vi "masternslave.vi"() -> ()   [LabVIEW 2020]
panel:
  in  "Requested Configuration (2: Query)":u32(ring)=2 items=["Off", "On", "Query"]
  out "Target Power Enabled?":bool
  in  "stop":bool
  out "Actual Bitrate kHz":i32=1000
  in  "Requested Bitrate kHz (1000)":i32=1000 min=0 max=50000
  out "Unique Ids":u32[](array[numeric])
  out "Data In":u8[](array[numeric]) format="%.0x"
  out "Total Shifted Out":i32
  in  "Max Bytes to Retrieve (256)":u32=256 min=1
  out "Batch Length":i32
  in  "Data Out (none)":u32[](array[numeric]) format="%.0x"
  in  "Output Enable (on)":bool=TRUE
  out "Ports":u16[](array[numeric])
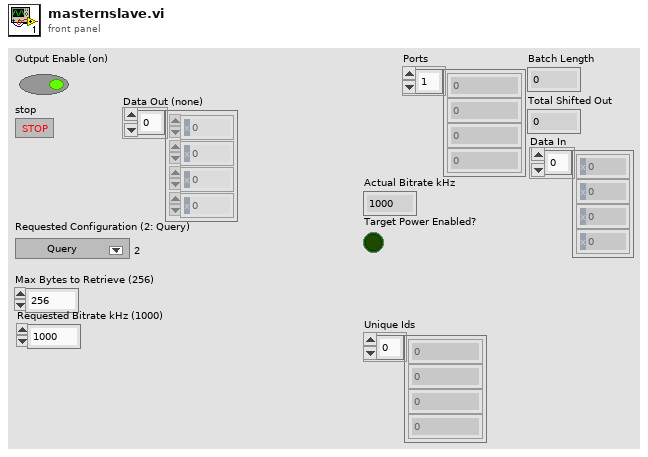
[diagram p1: front panel]
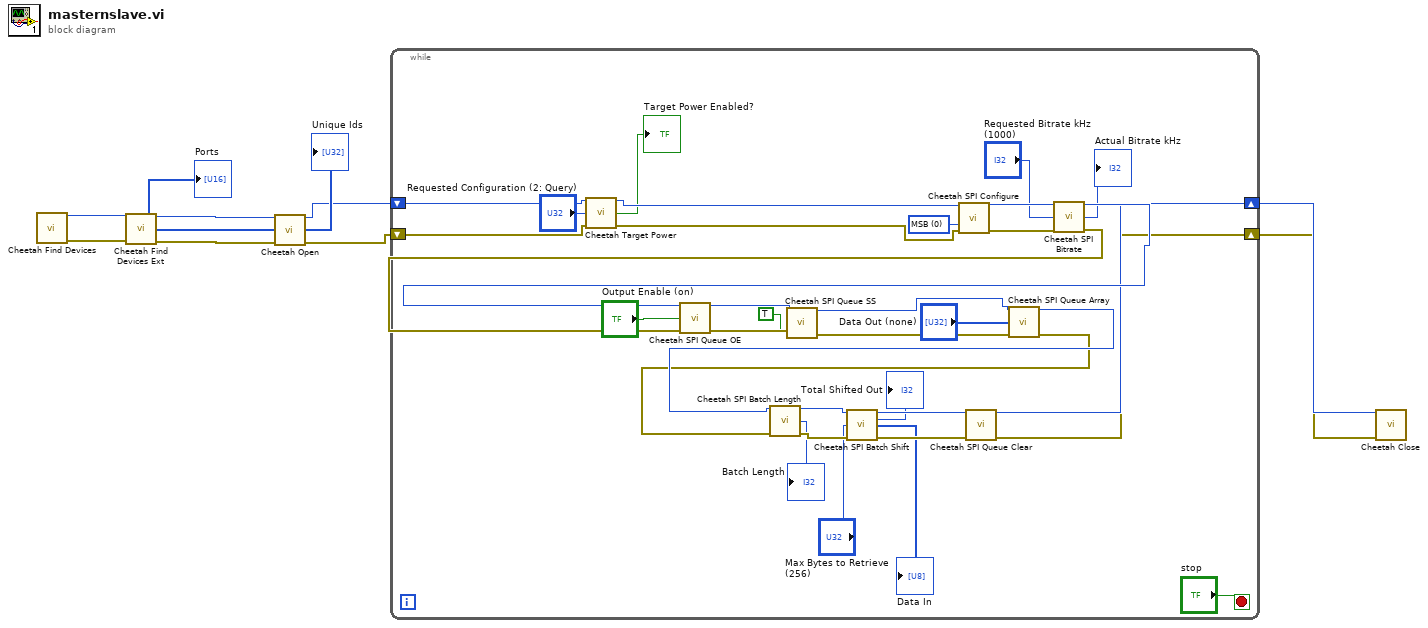
[diagram p0: block diagram]
diagram:
  n1 = call <instrlib>:"Cheetah Find Devices.vi"() -> ("Number found"=w10:i32, "error out"=w9:errorcluster)  [unwired: 13 in, 1 out]
  n2 = call <instrlib>:"Cheetah Find Devices Ext.vi"("Number of Ports (4)"=w10, "error in (no error)"=w9) -> ("Number found"=w8:i32, "Ports"=→"Ports":u16[], "Unique Ids"=→"Unique Ids":u32[], "error out"=w5:errorcluster)  [unwired: 10 in]
  n3 = call <instrlib>:"Cheetah Open.vi"("Port Number (0)"=w8, "error in (no error)"=w5) -> ("Cheetah Handle"=w1:i32, "error out"=w2:errorcluster)  [unwired: 12 in]
  n4 = while {
    shift-right: [w27] -> w7
    shift-left: w1 -> [w14]
    shift-right: [w26] -> w6
    shift-left: w2 -> [w15]
    stop <- "stop" stop-if-true
    w43 = 0 items=["MSB", "LSB"] ("Bitorder (0: MSB)")
    n5 = call <instrlib>:"Cheetah Target Power.vi"("Cheetah Handle"=w14, "Requested Configuration (2: Query)"="Requested Configuration (2: Query)", "error in (no error)"=w15) -> ("dup Cheetah Handle"=w13:i32, "Target Power Enabled?"=→"Target Power Enabled?":bool, "error out"=w16:errorcluster)  [unwired: 10 in]
    n6 = call <instrlib>:"Cheetah SPI Configure.vi"("Cheetah Handle"=w13, "Bitorder (0: MSB)"=w43, "error in (no error)"=w16) -> ("dup Cheetah Handle"=w42:i32, "error out"=w41:errorcluster)  [unwired: 11 in]
    n7 = call <instrlib>:"Cheetah SPI Bitrate.vi"("Cheetah Handle"=w42, "Requested Bitrate kHz (1000)"="Requested Bitrate kHz (1000)", "error in (no error)"=w41) -> ("dup Cheetah Handle"=w40:i32, "Actual Bitrate kHz"=→"Actual Bitrate kHz":i32, "error out"=w39:errorcluster)  [unwired: 10 in]
    n8 = call <instrlib>:"Cheetah SPI Queue OE.vi"("Cheetah Handle"=w40, "Output Enable (on)"="Output Enable (on)", "error in (no error)"=w39) -> ("dup Cheetah Handle"=w38:i32, "error out"=w37:errorcluster)  [unwired: 11 in]
    n9 = call <instrlib>:"Cheetah SPI Queue SS.vi"("Cheetah Handle"=w38, "SS2 Assert? (True)"=TRUE, "error in (no error)"=w37) -> ("dup Cheetah Handle"=w22:i32, "error out"=w23:errorcluster)  [unwired: 11 in]
    n10 = call <instrlib>:"Cheetah SPI Queue Array.vi"("Cheetah Handle"=w22, "Data Out (none)"="Data Out (none)", "error in (no error)"=w23) -> ("dup Cheetah Handle"=w21:i32, "error out"=w20:errorcluster)  [unwired: 11 in]
    n11 = call <instrlib>:"Cheetah SPI Batch Length.vi"("Cheetah Handle"=w21, "error in (no error)"=w20) -> ("dup Cheetah Handle"=w34:i32, "Batch Length"=→"Batch Length":i32, "error out"=w33:errorcluster)  [unwired: 11 in]
    n12 = call <instrlib>:"Cheetah SPI Batch Shift.vi"("Cheetah Handle"=w34, "Max Bytes to Retrieve (256)"="Max Bytes to Retrieve (256)", "error in (no error)"=w33) -> ("dup Cheetah Handle"=w36:i32, "Total Shifted Out"=→"Total Shifted Out":i32, "Data In"=→"Data In":u8[], "error out"=w35:errorcluster)  [unwired: 9 in]
    n13 = call <instrlib>:"Cheetah SPI Queue Clear.vi"("Cheetah Handle"=w36, "error in (no error)"=w35) -> ("dup Cheetah Handle"=w27:i32, "error out"=w26:errorcluster)  [unwired: 12 in]
  }
  n14 = call <instrlib>:"Cheetah Close.vi"("Cheetah Handle"=w7, "error in (no error)"=w6) -> ()  [unwired: 12 in, 2 out]
